vi "U16ToType.vi"(4 "U16 In":u16) -> (1 "Type out":T1=enum."RATIONAL")   [LabVIEW 2014, in "LAVA TIFF File Reader.lvlib"]
uses:
  LAVA TIFF File Reader.lvlib
  TypeDefs/FieldTypes.ctl
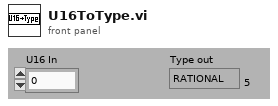
[diagram p1: front panel]
types:
  T1 = typedef "LAVA TIFF File Reader.lvlib/FieldTypes.ctl" = enum16{"NULL", "U8", "ASCII7", "U16", "U32", "RATIONAL", "SByte(I8)", "Undef(8Bit)", "I16", "I32", "SRat(4B:4B)", "SGL(4Byte)", "DBL(8Byte)"}
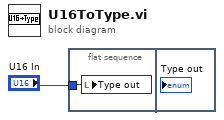
[diagram p0: block diagram]
diagram:
  n1 = flat-sequence {
    tunnel: "U16 In" -> [w2]
    frame #0 {
      n2 = local write "Type out"(w2) -> ()
    }
    frame #1 {
    }
  }
